vi "ConnectionQuality.vi"(9 "Oracle Timestamp":timestamp, 11 "Error?":bool) -> (1 "Last Update":timestamp, 3 "Connection Quality":dbl)   [LabVIEW 2017, in "Client.lvlib" / "CommsServer.lvlib"]
uses:
  CommsServer.lvlib
  <vilib>/ptbypt/NI_PtbyPt.lvlib
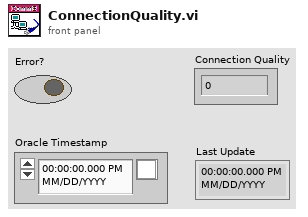
[diagram p1: front panel]
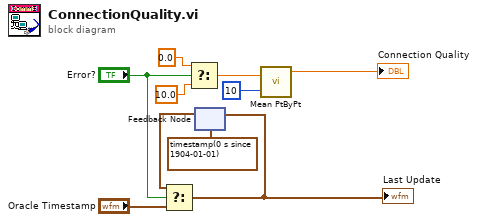
[diagram p0: block diagram]
diagram:
  n1 = Select(t=0.0, s="Error?", f=10.0) -> (s? t:f=w7:dbl)
  n2 = feedback #1(timestamp(0 s since 1904-01-01) ("seconds since 1Jan1904")) -> (w4:timestamp)
  n3 = Select(t=w4, s="Error?", f="Oracle Timestamp") -> (s? t:f=w5:timestamp)
  "Last Update" <- w5
  n4 = feedback-in #1(w5) -> ()
  n5 = call <vilib>:"Mean PtByPt.vi"("x"=w7, "sample length"=10) -> ("mean"=→"Connection Quality":dbl)  [unwired: 2 in, 1 out]
